vi "CheckModel.vi"(8 "Error In":errorcluster) -> (0 "Error Out":errorcluster, 2 "TestResult":bool, 3 "TestData":string)   [LabVIEW 2013]
uses:
  MainProgram/Control/Buffer.vi
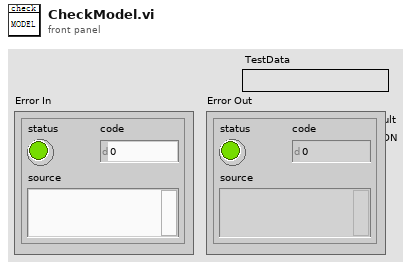
[diagram p1: front panel]
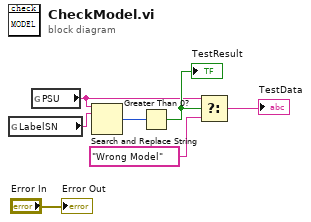
[diagram p0: block diagram]
diagram:
  n1 = global read "Buffer.vi" "LabelSN"() -> (w3:string)
  n2 = global read "Buffer.vi" "PSU"() -> (w2:string)
  n3 = Search and Replace String(input string=w2, search string=w3) -> (number of replacements=w6:i32)  [unwired: 6 in, 3 out]
  n4 = Greater Than 0?(x=w6) -> (x > 0?=w5:bool)
  "TestResult" <- w5
  n5 = Select(t=w2, s=w5, f="Wrong Model") -> (s? t:f=→"TestData":string)
  "Error Out" <- "Error In"
